vi "ExportToExcel.vi"(6 "Comments":string="Comment Thread", 7 "Channel Names":string[](array[string]), 8 "error in (no error)":errorcluster, 9 "Raw Data":dbl[][][](array[numeric]), 10 "Processed Data":dbl[][](array[numeric]), 11 "File Name":path) -> (0 "error out":errorcluster)   [LabVIEW 2009]
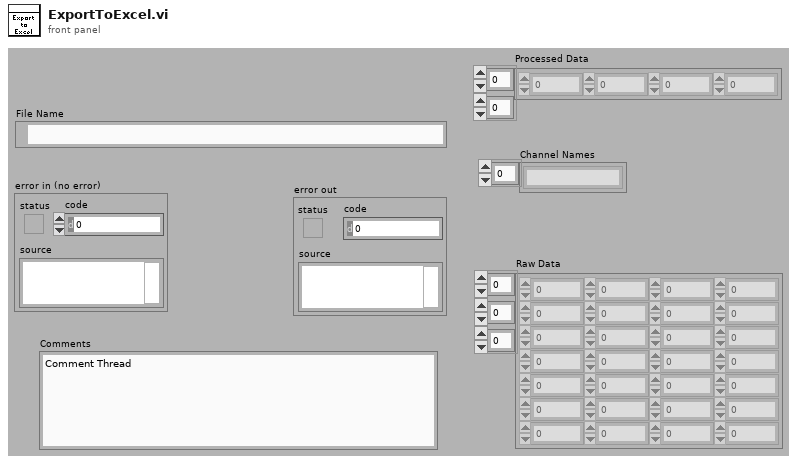
[diagram p1: front panel]
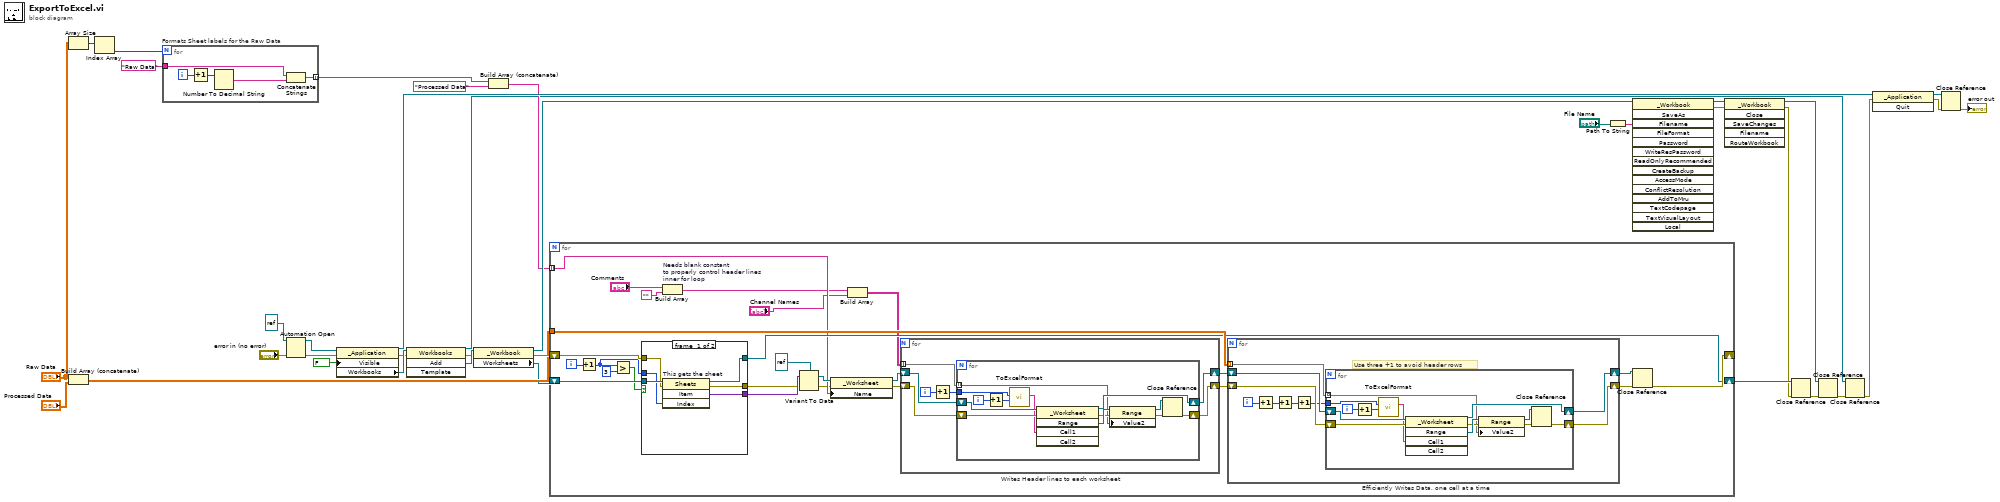
[diagram p0: block diagram]
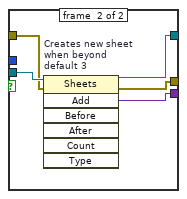
[diagram p2: hidden frame]
diagram:
  n1 = Array Size(array="Raw Data") -> (size(s)=w13:i32[])
  n2 = Build Array (concatenate)("Raw Data", "Processed Data") -> (w16:dbl[][][])
  n3 = Index Array(array=w13) -> (element=w12:i32)  [unwired: 1 in]
  n4 = for "Formats Sheet labels for the Raw Data" {
    N: w12 -> [_]
    tunnel: "Raw Data" -> [w41]
    tunnel: [w39] -> w10 mode=indexing
    i -> [w38]
    n5 = Increment(x=w38) -> (x+1=w37:i32)
    n6 = Number To Decimal String(number=w37) -> (decimal integer string=w40:string)  [unwired: 1 in]
    n7 = Concatenate Strings(w41, w40) -> (w39:string)
  }
  n8 = Automation Open(error in (no error)="error in (no error)", Automation Refnum=refnum<k7> refnum ("Excel Application")) -> (Automation Refnum=w33:refnum<k7>, error out=w34:errorcluster)  [unwired: 2 in]
  n9 = property class="_Application"(reference=w33, error in=w34, "Visible"=FALSE) -> (reference out=w23:refnum<k7>, error out=w29:errorcluster, "Workbooks"=w31:refnum<k7>)
  n10 = invoke class="Workbooks" method="Add"(reference=w31, error in=w29) -> (reference out=w7:refnum<k7>, error out=w28:errorcluster, "Add"=w30:refnum<k7>)  [unwired: 2 in, 1 out]
  n11 = property class="_Workbook"(reference=w30, error in=w28) -> (reference out=w26:refnum<k7>, error out=w27:errorcluster, "Worksheets"=w15:refnum<k7>)
  n12 = Build Array (concatenate)(w10, "Processed Data") -> (w14:string[])
  n13 = for {
    shift-right: [w60] -> _
    shift-left: w27 -> [w64]
    shift-right: [w57] -> w8
    shift-left: w15 -> [w67]
    tunnel: w16 -> [w58]
    tunnel: w14 -> [w55] mode=indexing
    i -> [w59]
    n14 = Increment(x=w59) -> (x+1=w52:i32)
    n15 = Greater?(x=w52, y=3) -> (0:w53:bool)
    n16 = case shown="False" w53 {
      tunnel: w67 -> [w93 w98]
      tunnel: [w92 w96] -> w66
      tunnel: w64 -> [w91 w97]
      tunnel: [w90 w95] -> w63
      tunnel: w52 -> [w89 _]
      tunnel: [w88 w94] -> w57
      frame #0 {
        n17 = invoke on="This gets the sheet" class="Sheets" method="Item"(reference=w93, error in=w91, "Index"=w89) -> (reference out=w88:refnum<k7>, error out=w90:errorcluster, "Item"=w92:variant)  [unwired: 1 in, 1 out]
      }
      frame #1 {
        n18 = invoke on="Creates new sheet\nwhen beyond\ndefault 3" class="Sheets" method="Add"(reference=w98, error in=w97) -> (reference out=w94:refnum<k7>, error out=w95:errorcluster, "Add"=w96:variant)  [unwired: 5 in, 4 out]
      }
    }
    n19 = Build Array "Needs blank constant\nto properly control header lines\ninner for loop"("Comments", "") -> (w43:string[])
    n20 = Variant To Data(error in=w63, Variant=w66, type=refnum<k7> refnum ("reference")) -> (error out=w54:errorcluster, data=w56:refnum<k7>)
    n21 = property class="_Worksheet"(reference=w56, error in=w54, "Name"=w55) -> (reference out=w49:refnum<k7>, error out=w48:errorcluster)
    n22 = Build Array(w43, "Channel Names") -> (w50:string[][])
    n23 = for "Writes Header lines to each worksheet" {
      shift-right: [w70] -> w46
      shift-left: w48 -> [w73]
      shift-right: [w71] -> w47
      shift-left: w49 -> [w74]
      tunnel: w50 -> [w72] mode=indexing
      i -> [w69]
      n24 = Increment(x=w69) -> (x+1=w68:i32)
      n25 = for {
        shift-right: [w81] -> w70
        shift-left: w73 -> [w84]
        shift-right: [w80] -> w71
        shift-left: w74 -> [w87]
        tunnel: w68 -> [w78]
        tunnel: w72 -> [w77] mode=indexing
        i -> [w76]
        n26 = Increment(x=w76) -> (x+1=w75:i32)
        n27 = call "ToExcelFormat.vi"("Column"=w75, "Row"=w78) -> ("Output String"=w79:string)  [unwired: 9 in]
        n28 = invoke class="_Worksheet" method="Range"(reference=w87, error in=w84, "Cell1"=w79) -> (reference out=w80:refnum<k7>, error out=w83:errorcluster, "Range"=w86:refnum<k7>)  [unwired: 2 in, 2 out]
        n29 = property class="Range"(reference=w86, error in=w83, "Value2"=w77) -> (reference out=w85:refnum<k7>, error out=w82:errorcluster)
        n30 = Close Reference(reference=w85, error in (no error)=w82) -> (error out=w81:errorcluster)
      }
    }
    n31 = for "Efficiently Writes Data, one cell at a time" {
      shift-right: [w105] -> w62
      shift-left: w46 -> [w106]
      shift-right: [w104] -> w61
      shift-left: w47 -> [w107]
      tunnel: w58 -> [w103] mode=indexing
      i -> [w102]
      # "Use three +1 to avoid header rows"
      n32 = Increment(x=w102) -> (x+1=w101:i32)
      n33 = Increment(x=w101) -> (x+1=w100:i32)
      n34 = Increment(x=w100) -> (x+1=w99:i32)
      n35 = for {
        shift-right: [w114] -> w105
        shift-left: w106 -> [w117]
        shift-right: [w113] -> w104
        shift-left: w107 -> [w120]
        tunnel: w99 -> [w111]
        tunnel: w103 -> [w110] mode=indexing
        i -> [w109]
        n36 = Increment(x=w109) -> (x+1=w108:i32)
        n37 = call "ToExcelFormat.vi"("Column"=w108, "Row"=w111) -> ("Output String"=w112:string)  [unwired: 9 in]
        n38 = invoke class="_Worksheet" method="Range"(reference=w120, error in=w117, "Cell1"=w112) -> (reference out=w113:refnum<k7>, error out=w116:errorcluster, "Range"=w119:refnum<k7>)  [unwired: 2 in, 2 out]
        n39 = property class="Range"(reference=w119, error in=w116, "Value2"=w110) -> (reference out=w118:refnum<k7>, error out=w115:errorcluster)
        n40 = Close Reference(reference=w118, error in (no error)=w115) -> (error out=w114:errorcluster)
      }
    }
    n41 = Close Reference(reference=w61, error in (no error)=w62) -> (error out=w60:errorcluster)
  }
  n42 = Path To String(path="File Name") -> (string=w17:string)
  n43 = invoke class="_Workbook" method="SaveAs"(reference=w26, "Filename"=w17) -> (reference out=w25:refnum<k7>, error out=w24:errorcluster)  [unwired: 13 in, 13 out]
  n44 = invoke class="_Workbook" method="Close"(reference=w25, error in=w24) -> (reference out=w22:refnum<k7>, error out=w4:errorcluster)  [unwired: 4 in, 4 out]
  n45 = Close Reference(reference=w8, error in (no error)=w4) -> (error out=w3:errorcluster)
  n46 = Close Reference(reference=w22, error in (no error)=w3) -> (error out=w6:errorcluster)
  n47 = Close Reference(reference=w7, error in (no error)=w6) -> (error out=w5:errorcluster)
  n48 = invoke class="_Application" method="Quit"(reference=w23, error in=w5) -> (reference out=w20:refnum<k7>, error out=w21:errorcluster)  [unwired: 1 in, 1 out]
  n49 = Close Reference(reference=w20, error in (no error)=w21) -> (error out=→"error out":errorcluster)
